vi "Kinect Offset Image To Base Of Contour.vi"(0 "Image In":T1, 5 "Spine Contour":i32[](array[numeric]), 7 "Butt Position (pixels from left of image)":i32=10, 9 "Butt Threshold":dbl=100.0) -> (4 "Image Out":T1)   [LabVIEW 2011]
uses:
  <vilib>/vision/Image Controls.llb/IMAQ Image.ctl
  <vilib>/Analysis/NI_AALPro.lvlib
  <vilib>/vision/NI_Vision_Development_Module.lvlib
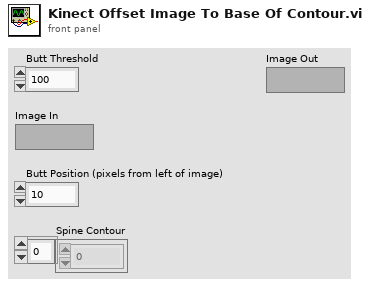
[diagram p1: front panel]
types:
  T1 = typedef "IMAQ Image.ctl" = refnum<image>
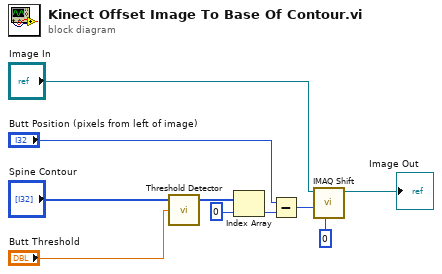
[diagram p0: block diagram]
diagram:
  n1 = call <vilib>:"Threshold Detector.vi"("threshold"="Butt Threshold", "X"="Spine Contour") -> ("Indices"=w2:i32[])  [unwired: 1 in, 2 out]
  n2 = Index Array(array=w2, index=0) -> (element=w5:i32)
  n3 = Subtract(x="Butt Position (pixels from left of image)", y=w5) -> (x-y=w1:i32)
  n4 = call "IMAQ Shift"("YOffset"=0, "XOffset"=w1, "Image Src"="Image In") -> ("Image Dst Out"=→"Image Out":T1)  [unwired: 7 in, 1 out]
